vi "Channels to Hex.vi"(5 "RF Chip1 Enable":bool, 7 "RF Chip0 Enable":bool, 10 "RF Chip0 Channel":u8, 11 "RF Chip1 Channel":u8) -> (3 "Command":u8[](array[numeric]))   [LabVIEW 2015]
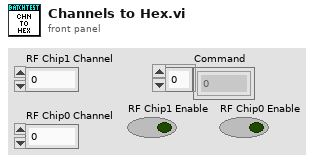
[diagram p1: front panel]
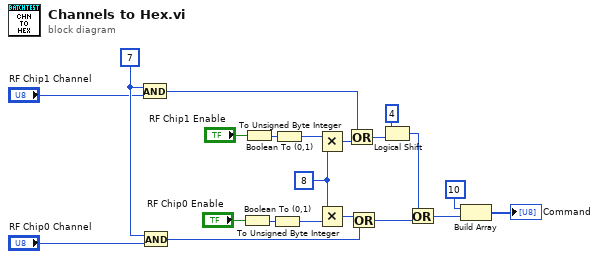
[diagram p0: block diagram]
diagram:
  w18 = u8 8
  w20 = u8 7
  n1 = And(x=w20, y="RF Chip1 Channel") -> (x .and. y?=w17:u8)
  n2 = And(x=w20, y="RF Chip0 Channel") -> (x .and. y?=w7:u8)
  n3 = Boolean To (0,1)(Boolean="RF Chip0 Enable") -> (0, 1=w13:i16)
  n4 = Boolean To (0,1)(Boolean="RF Chip1 Enable") -> (0, 1=w9:i16)
  n5 = To Unsigned Byte Integer(number=w13) -> (unsigned 8bit integer=w19:u8)
  n6 = To Unsigned Byte Integer(number=w9) -> (unsigned 8bit integer=w11:u8)
  n7 = Multiply(x=w11, y=w18) -> (x*y=w16:u8)
  n8 = Multiply(x=w18, y=w19) -> (x*y=w15:u8)
  n9 = Or(x=w17, y=w16) -> (x .or. y?=w12:u8)
  n10 = Or(x=w15, y=w7) -> (x .or. y?=w21:u8)
  n11 = Logical Shift(y=i8 4, x=w12) -> (x << y=w5:u8)
  n12 = Or(x=w5, y=w21) -> (x .or. y?=w4:u8)
  n13 = Build Array(u8 10, w4) -> (→"Command":u8[])
